vi "GetInterleavingSynx.vi"(8 "error in (no error)":errorcluster, 11 "clEvtReportArrayIn":T1 {"Synx" format="%#_4g"}) -> (0 "error out":errorcluster, 3 "Synx":cdb[][](array[numeric]))   [LabVIEW 2017, in "AppPlugins.lvlib" / "LSEPlugin.lvclass"]
uses:
  LSEPlugin.lvclass
  EventPlugins/EventPluginBaseClass/TypeDefs/clEvtReportArray.ctl
  EventPlugins/EventPluginBaseClass/TypeDefs/clEvtReport.ctl
  EventPlugins/EventPluginBaseClass/EventPluginBaseClass.lvclass
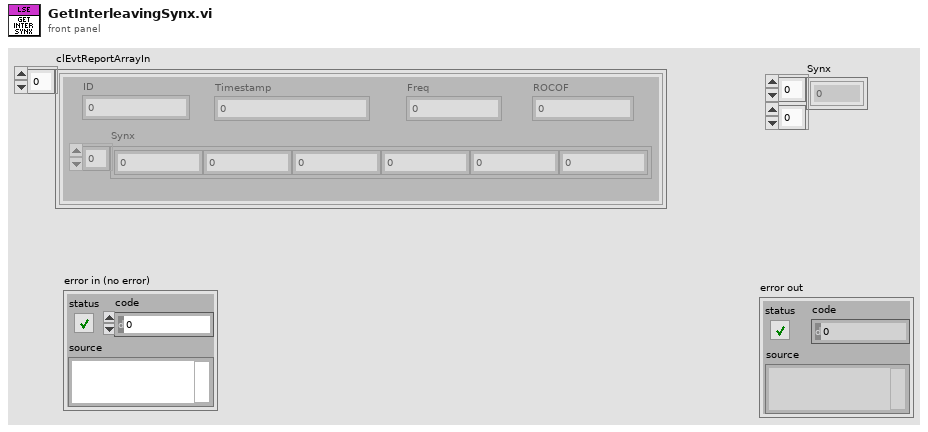
[diagram p1: front panel]
types:
  T1 = typedef "EventPlugins.lvlib/EventPluginBaseClass.lvclass/clEvtReportArray.ctl" = T2[]
  T2 = typedef "EventPlugins.lvlib/EventPluginBaseClass.lvclass/clEvtReport.ctl" = cluster{"Timestamp":dbl, "Synx":cdb[], "Freq":dbl, "ROCOF":dbl, "ID":i16}
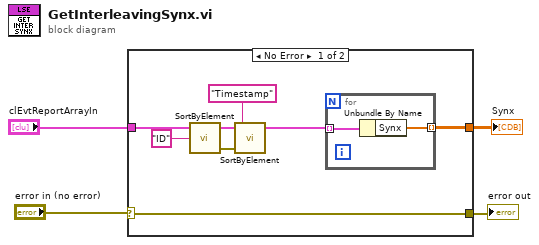
[diagram p0: block diagram]
diagram:
  n1 = case shown="No Error" "error in (no error)" {
    selector: "error in (no error)" -> [w5 w15]
    tunnel: "clEvtReportArrayIn" -> [w7 _]
    tunnel: [w6 _] -> w3
    tunnel: [w5 w15] -> w1
    frame No Error {
      n2 = call "SortByElement.vi"("String"="ID", "clEvtReportArrayIn"=w7) -> ("error out"=w8:errorcluster, "clEvtReportArrayOut"=w11:T1)  [unwired: 2 in]
      n3 = call "SortByElement.vi"("error in (no error)"=w8, "String"="Timestamp", "clEvtReportArrayIn"=w11) -> ("clEvtReportArrayOut"=w9:T1)  [unwired: 1 in, 1 out]
      n4 = for {
        tunnel: w9 -> [w14] mode=indexing
        tunnel: [w13] -> w6 mode=indexing
        n5 = Unbundle By Name(w14) -> ("Synx"=w13:cdb[])
      }
    }
    frame Error {
    }
  }
  "Synx" <- w3
  "error out" <- w1
